vi "State Actor Destroy.vi"(7 "Self Actor in":refnum<class "Self Actor.lvclass">, 11 "Self Actor State in":refnum<class "Self Actor State.lvclass">) -> (0 "error out":errorcluster)   [LabVIEW 2021, in "LVCAM.lvlib" / "Self Actor State.lvclass"]
uses:
  Self Actor State.lvclass
  Self Actor/Self Actor.lvclass
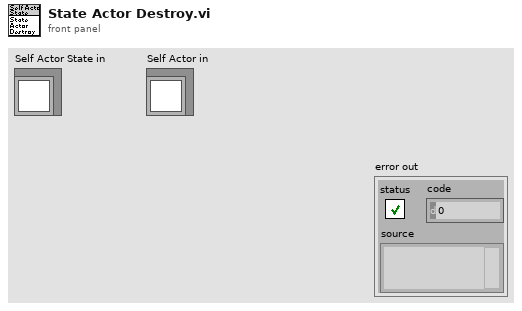
[diagram p1: front panel]
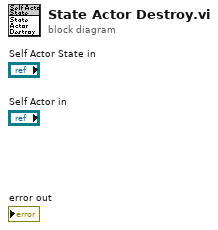
[diagram p0: block diagram]
diagram:
